vi "описание ошибки.vi"(11 "Numeric":dbl) -> (0 "String 2":string, 3 "String":string)   [LabVIEW 2016, in "Library.lvlib"]
uses:
  Granule-2000AT/PC/Library.lvlib
panel:
  out "floor(x/y)":dbl
  out "x-y*floor(x/y)":dbl
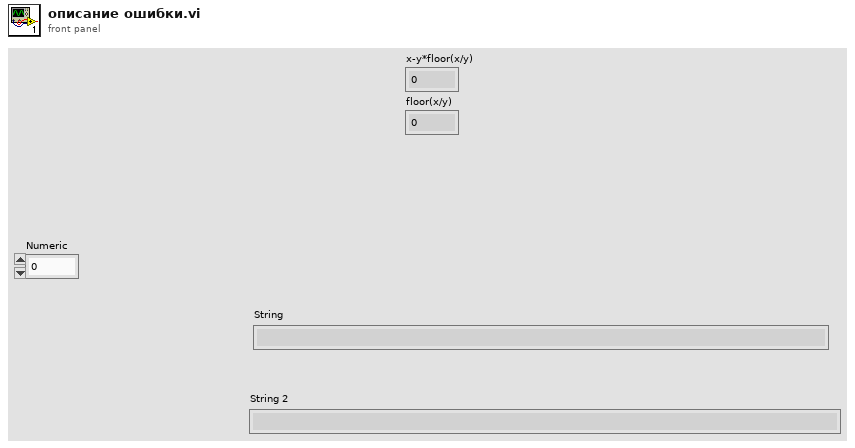
[diagram p1: front panel]
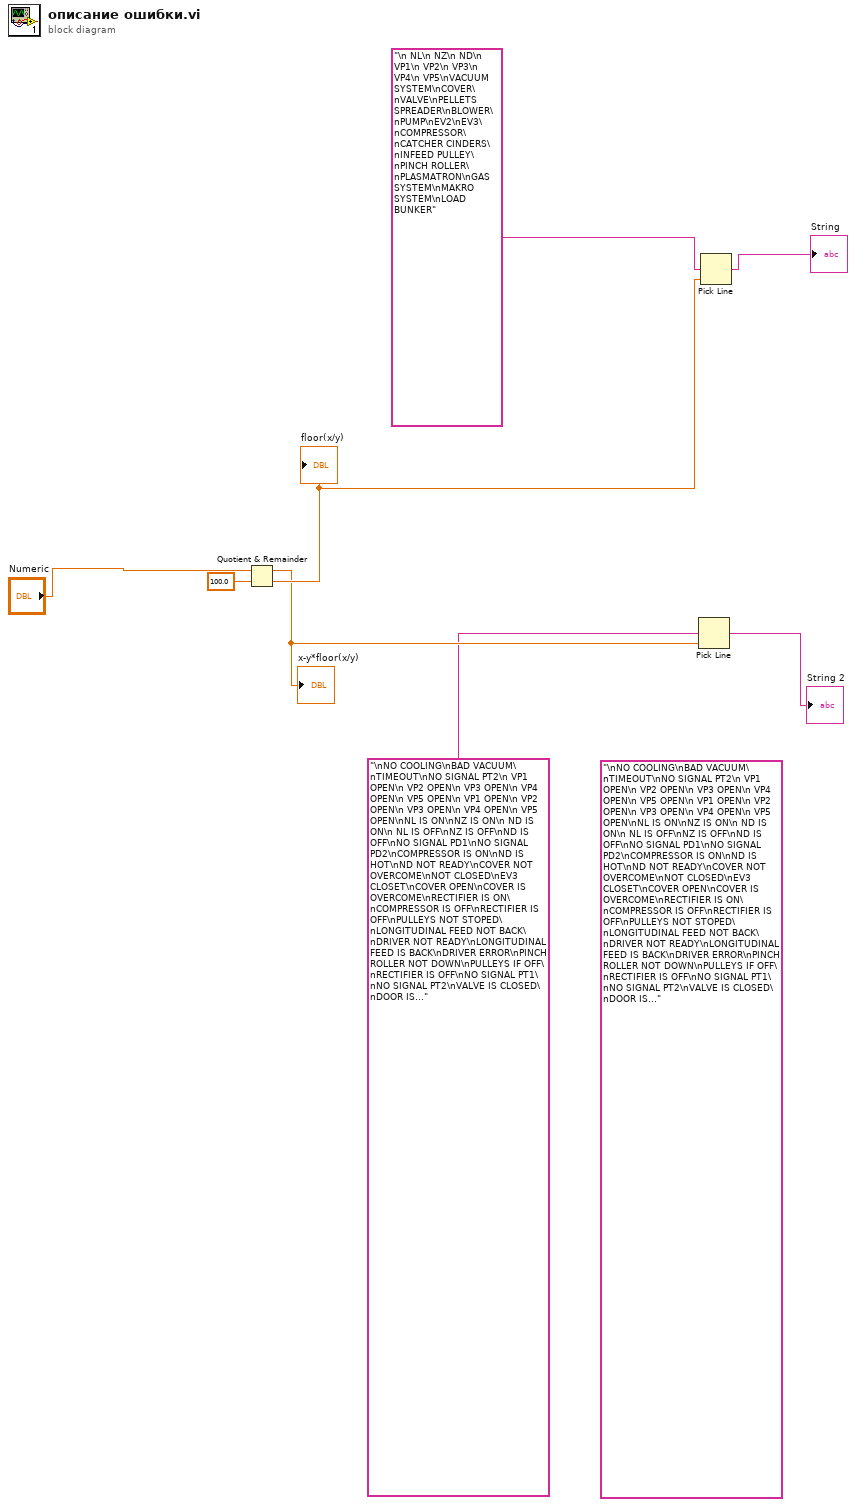
[diagram p0: block diagram]
diagram:
  (unwired) "\nNO COOLING\nBAD VACUUM\nTIMEOUT\nNO SIGNAL PT2\n VP1 OPEN\n VP2 OPEN\n VP3 OPEN\n VP4 OPEN\n VP5 OPEN\n VP1 OPEN\n VP2 OPEN\n VP3 OPEN\n VP4 OPEN\n VP5 OPEN\nNL IS ON\nNZ IS ON\n ND IS ON\n NL IS OFF\nNZ IS OFF\nND IS OFF\nNO SIGNAL PD1\nNO SIGNAL PD2\nCOMPRESSOR IS ON\nND IS HOT\nND NOT READY\nCOVER NOT OVERCOME\nNOT CLOSED\nEV3 CLOSET\nCOVER OPEN\nCOVER IS OVERCOME\nRECTIFIER IS ON\nCOMPRESSOR IS OFF\nRECTIFIER IS OFF\nPULLEYS NOT STOPED\nLONGITUDINAL FEED NOT BACK\nDRIVER NOT READY\nLONGITUDINAL FEED IS BACK\nDRIVER ERROR\nPINCH ROLLER NOT DOWN\nPULLEYS IF OFF\nRECTIFIER IS OFF\nNO SIGNAL PT1\nNO SIGNAL PT2\nVALVE IS CLOSED\nDOOR IS OPEN\nDOOR IS CLOSED\nDOOR IS PRESSED\nDOOR IS OVERCOME"
  n1 = Quotient & Remainder(x="Numeric", y=100.0) -> (x-y*floor(x/y)=w3:dbl, floor(x/y)=w5:dbl)
  "x-y*floor(x/y)" <- w3
  "floor(x/y)" <- w5
  n2 = Pick Line(multi-line string="\nNO COOLING\nBAD VACUUM\nTIMEOUT\nNO SIGNAL PT2\n VP1 OPEN\n VP2 OPEN\n VP3 OPEN\n VP4 OPEN\n VP5 OPEN\n VP1 OPEN\n VP2 OPEN\n VP3 OPEN\n VP4 OPEN\n VP5 OPEN\nNL IS ON\nNZ IS ON\n ND IS ON\n NL IS OFF\nNZ IS OFF\nND IS OFF\nNO SIGNAL PD1\nNO SIGNAL PD2\nCOMPRESSOR IS ON\nND IS HOT\nND NOT READY\nCOVER NOT OVERCOME\nNOT CLOSED\nEV3 CLOSET\nCOVER OPEN\nCOVER IS OVERCOME\nRECTIFIER IS ON\nCOMPRESSOR IS OFF\nRECTIFIER IS OFF\nPULLEYS NOT STOPED\nLONGITUDINAL FEED NOT BACK\nDRIVER NOT READY\nLONGITUDINAL FEED IS BACK\nDRIVER ERROR\nPINCH ROLLER NOT DOWN\nPULLEYS IF OFF\nRECTIFIER IS OFF\nNO SIGNAL PT1\nNO SIGNAL PT2\nVALVE IS CLOSED\nDOOR IS OPEN\nDOOR IS CLOSED\nDOOR IS PRESSED\nDOOR IS OVERCOME", line index=w3) -> (output string=→"String 2":string)  [unwired: 1 in]
  n3 = Pick Line(multi-line string="\n NL\n NZ\n ND\n VP1\n VP2\n VP3\n VP4\n VP5\nVACUUM SYSTEM\nCOVER\nVALVE\nPELLETS SPREADER\nBLOWER\nPUMP\nEV2\nEV3\nCOMPRESSOR\nCATCHER CINDERS\nINFEED PULLEY\nPINCH ROLLER\nPLASMATRON\nGAS SYSTEM\nMAKRO SYSTEM\nLOAD BUNKER", line index=w5) -> (output string=→"String":string)  [unwired: 1 in]
